vi "流程写入.vi"(10 "简易流程路径":path, 11 "添加的路径":path caption="测试流程路径") -> ()   [LabVIEW 2016, in "斯坦道总氮.lvlib"]
uses:
  <vilib>/Utility/miscctls.llb/LVPointTypeDef.ctl
panel:
  in  "选项卡控件":enum32{"测试流程", "简易流程"}(tab)
  in  "一键写入":bool
  in  "量程下拉列表":enum16{"低量程", "高量程"}(ring)
  in  "测量模式":T1(ring)
  in  "简易流程":u16(ring)
  in  "一键写入 2":bool=TRUE
  in  "关闭":bool
  out "字符串":string
  in  "写入":bool
  in  "参数下拉列表":u16(ring)
  # "请选择要写入的流程"
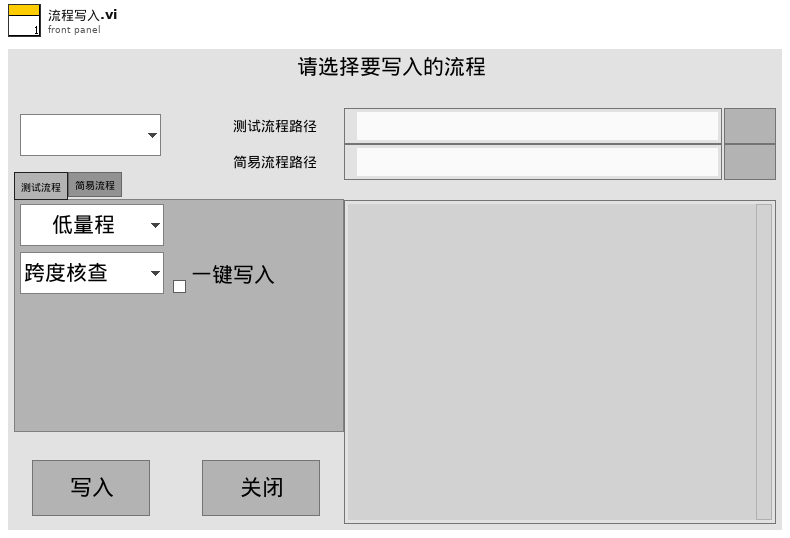
[diagram p1: front panel]
types:
  T1 = enum16{"跨度核查", "水样测量", "零点核查", "标样核查", "加标回收", "快捷测试", "空白校准", "标样校准"}
  T2 = typedef "LVPointTypeDef.ctl" = cluster{"Horizontal":i16, "Vertical":i16}
  T3 = typedef "LVStringsAndValuesArrayTypeDef_U16.ctl" = cluster{"String":string, "Value":u16}[]
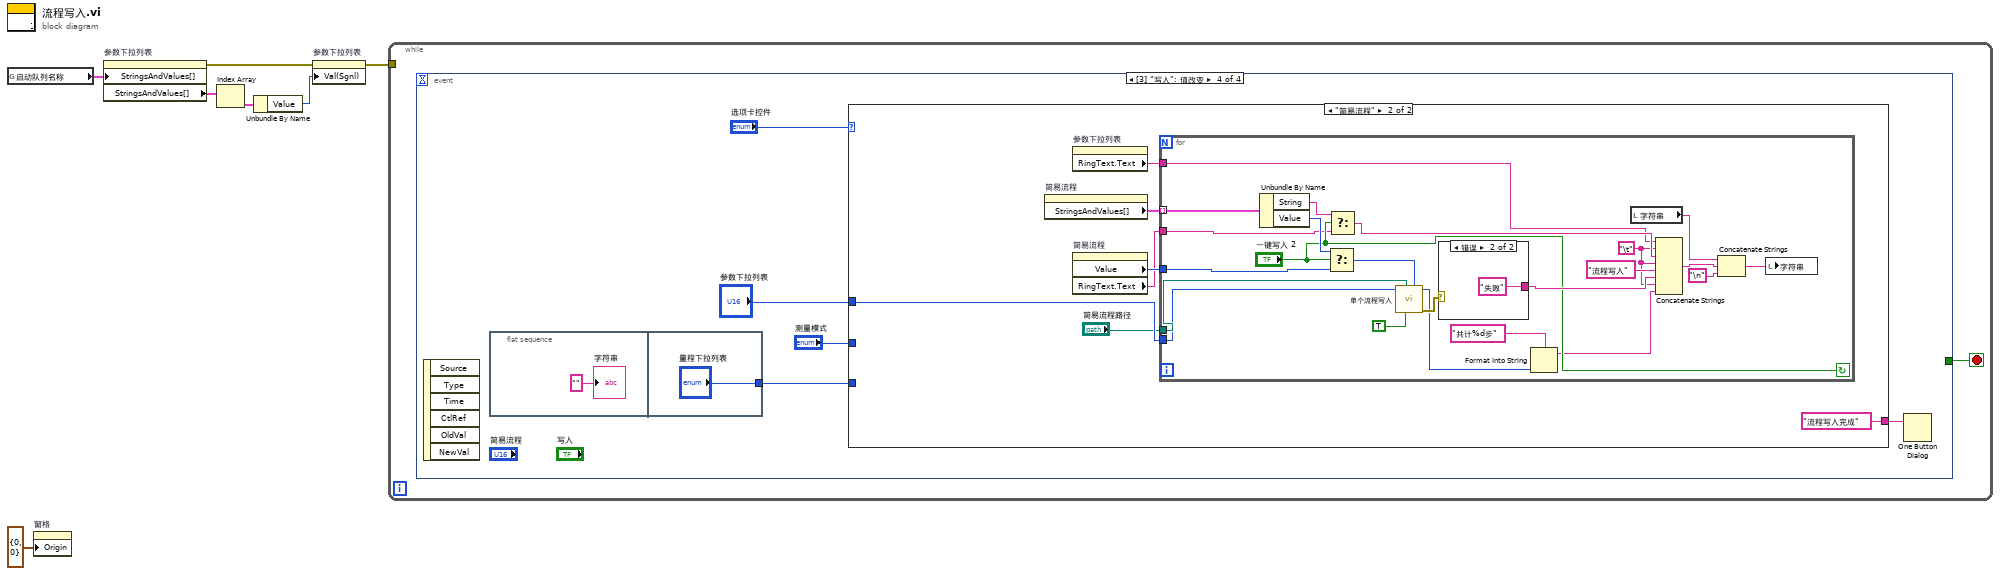
[diagram p0: block diagram]
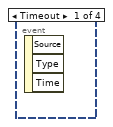
[diagram p2: hidden frame]
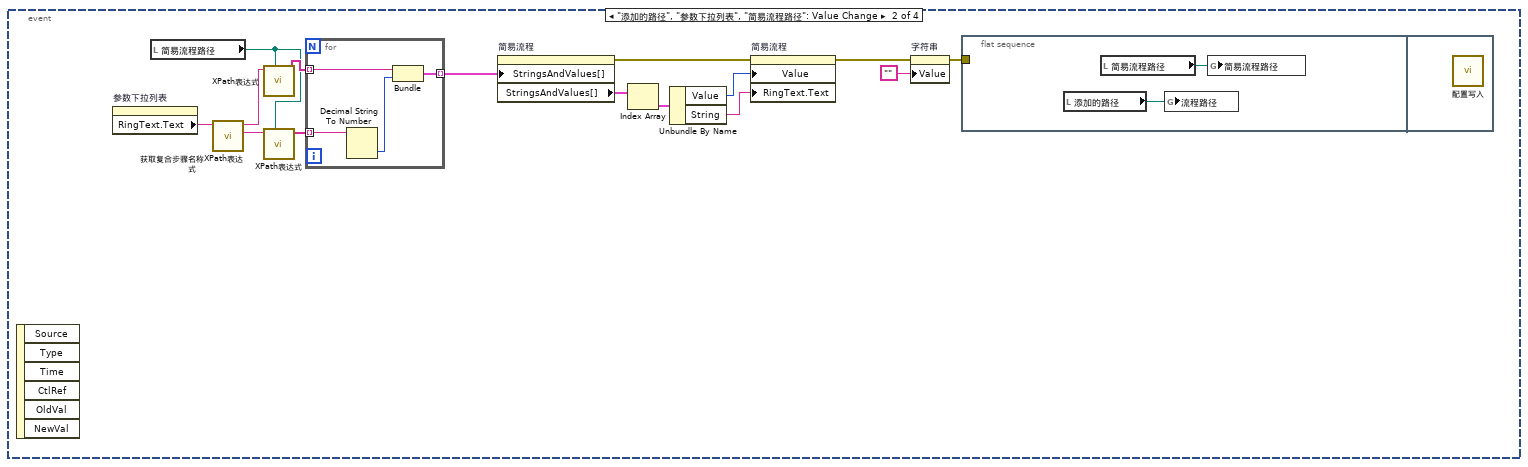
[diagram p3: hidden frame]
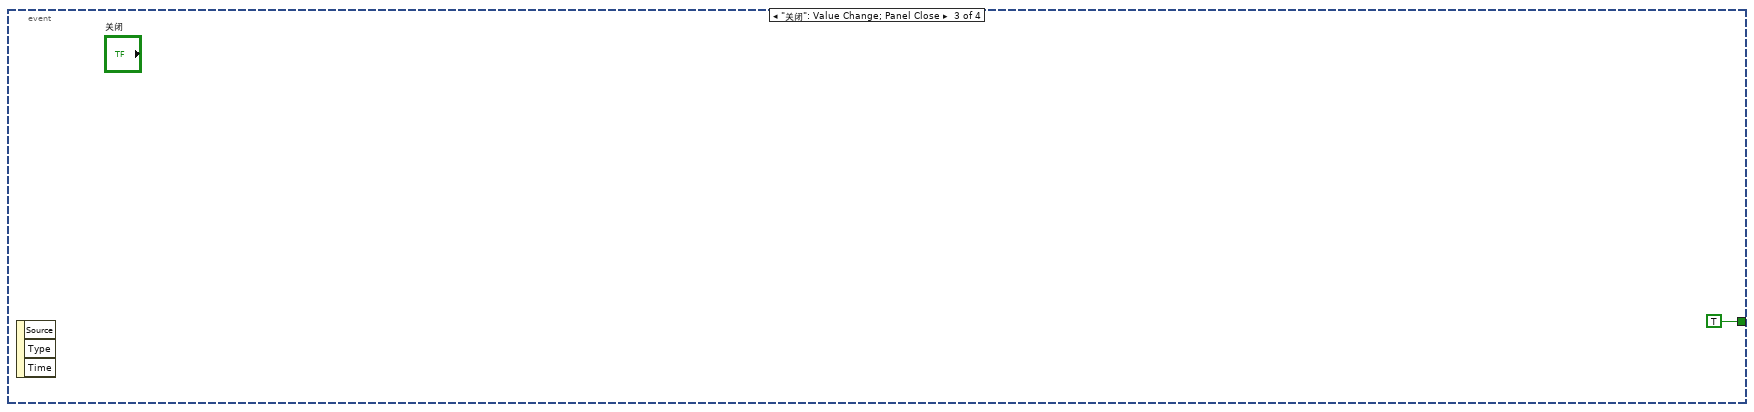
[diagram p4: hidden frame]
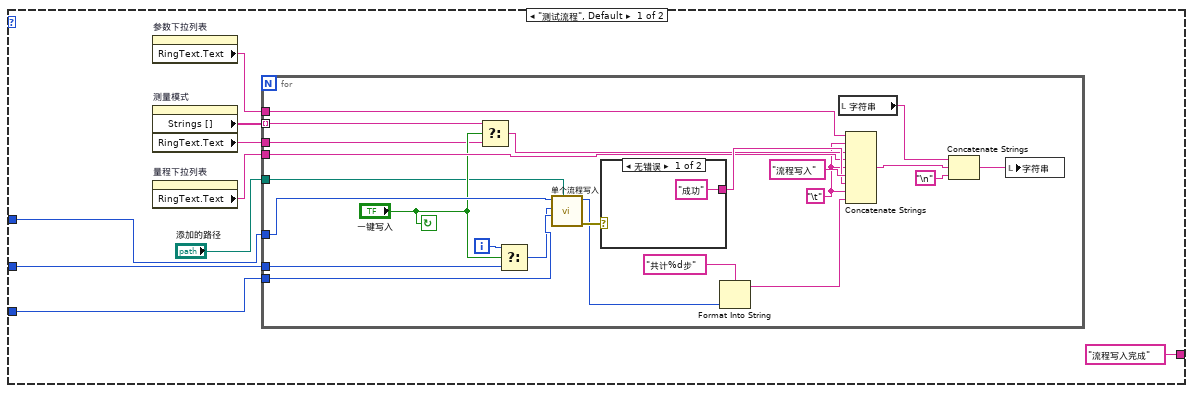
[diagram p5: hidden frame]
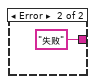
[diagram p6: hidden frame]
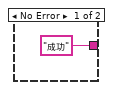
[diagram p7: hidden frame]
diagram:
  n1 = global read "总磷总氮断电保存全局变量.vi" "启动队列名称"() -> (w6:cluster{"String":string, "Value":u16}[])
  n2 = property on="窗格" class="Pane"("Origin"=T2 {"Horizontal"=0, "Vertical"=0} ("原点")) -> ()  [unwired: 2 in, 2 out]
  n3 = property on="参数下拉列表" class="Ring (严格)"("StringsAndValues[]"=w6) -> (error out=w5:errorcluster, "StringsAndValues[]"=w4:T3)  [unwired: 2 in, 1 out]
  n4 = Index Array(array=w4) -> (element=w3:cluster{"String":string, "Value":u16})  [unwired: 1 in]
  n5 = Unbundle By Name(w3) -> ("Value"=w2:u16)
  n6 = property on="参数下拉列表" class="Ring (严格)"(error in=w5, "Val(Sgnl)"=w2) -> (error out=w1:errorcluster)  [unwired: 1 in, 1 out]
  n7 = while {
    tunnel: w1 -> [_]
    stop <- w8 stop-if-true
    n8 = event shown="[3] \"写入\": 值改变" {
      selector: _ -> [_ _ _ _]
      dyn-events: _ -> [_ _ _ _]
      timeout: _ -> [_ _ _ _]
      tunnel: [_ _ TRUE _] -> w8
      event Timeout {
        n9 = event-data() -> ()  [unwired: 1 in, 3 out]
      }
      event "添加的路径", "参数下拉列表", "简易流程路径": Value Change {
        n10 = event-data() -> ()  [unwired: 1 in, 6 out]
        n11 = property on="参数下拉列表" class="Ring (严格)"() -> ("RingText.Text"=w22:string)  [unwired: 2 in, 2 out]
        n12 = local read "简易流程路径"() -> (w16:path)
        n13 = call "获取复合步骤名称XPath表达式.vi"("查询参数"=w22) -> ("FlowId"=w21:string, "name"=w23:string)  [unwired: 9 in]
        n14 = call "XPath表达式.vi"("添加的路径"=w16, "XPath expression"=w23) -> ("数组"=w20:string[])  [unwired: 9 in]
        n15 = call "XPath表达式.vi"("添加的路径"=w16, "XPath expression"=w21) -> ("数组"=w19:string[])  [unwired: 9 in]
        n16 = for {
          tunnel: w20 -> [w29] mode=indexing
          tunnel: w19 -> [w28] mode=indexing
          tunnel: [w26] -> w18 mode=indexing
          n17 = Decimal String To Number(string=w28) -> (number=w27:i32)  [unwired: 2 in, 1 out]
          n18 = Bundle("node text"=w29, w27) -> (w26:cluster{"node text":string, i32})  [unwired: 1 in]
        }
        n19 = property on="简易流程" class="Ring (严格)"("StringsAndValues[]"=w18) -> (error out=w15:errorcluster, "StringsAndValues[]"=w13:T3)  [unwired: 2 in, 1 out]
        n20 = Index Array(array=w13) -> (element=w12:cluster{"String":string, "Value":u16})  [unwired: 1 in]
        n21 = Unbundle By Name(w12) -> ("Value"=w11:u16, "String"=w9:string)
        n22 = property on="简易流程" class="Ring (严格)"(error in=w15, "Value"=w11, "RingText.Text"=w9) -> (error out=w14:errorcluster)  [unwired: 1 in, 1 out]
        n23 = property on="字符串" class="Str"(error in=w14, "Value"="") -> (error out=w10:errorcluster)  [unwired: 1 in, 1 out]
        n24 = flat-sequence {
          tunnel: w10 -> [_]
          frame #0 {
            n25 = local read "添加的路径"() -> (w24:path)
            n26 = local read "简易流程路径"() -> (w25:path)
            n27 = global write "总磷总氮断电保存全局变量.vi" "流程路径"(w24) -> ()
            n28 = global write "总磷总氮断电保存全局变量.vi" "简易流程路径"(w25) -> ()
          }
          frame #1 {
            n29 = call "配置写入.vi"() -> ()  [unwired: 11 in, 1 out]
          }
        }
      }
      event "关闭": Value Change; Panel Close {
        n30 = event-data() -> ()  [unwired: 1 in, 3 out]
      }
      event "写入": Value Change {
        n31 = event-data() -> ()  [unwired: 1 in, 6 out]
        n32 = flat-sequence {
          tunnel: ["量程下拉列表"] -> w34
          frame #0 {
            "字符串" <- ""
          }
          frame #1 {
          }
        }
        n33 = case shown="\"简易流程\"" "选项卡控件" {
          tunnel: "参数下拉列表" -> [w42 w76]
          tunnel: w34 -> [w43 _]
          tunnel: ["流程写入完成" ("消息") "流程写入完成" ("消息")] -> w32
          tunnel: "测量模式" -> [w40 _]
          frame "测试流程", Default {
            n34 = property on="参数下拉列表" class="Ring (严格)"() -> ("RingText.Text"=w37:string)  [unwired: 2 in, 2 out]
            n35 = property on="测量模式" class="Enum (严格)"() -> ("Strings []"=w41:string[], "RingText.Text"=w38:string)  [unwired: 2 in, 2 out]
            n36 = property on="量程下拉列表" class="Enum (严格)"() -> ("RingText.Text"=w39:string)  [unwired: 2 in, 2 out]
            n37 = for {
              tunnel: w43 -> [w60]
              tunnel: w42 -> [w58]
              tunnel: w41 -> [w53] mode=indexing
              tunnel: w40 -> [w57]
              tunnel: w39 -> [w55]
              tunnel: w38 -> [w52]
              tunnel: "添加的路径" -> [w50]
              tunnel: w37 -> [w49]
              i -> [w59]
              stop <- "一键写入" continue-if-true
              w45 = "\t"
              n38 = Select(t=w53, s="一键写入", f=w52) -> (s? t:f=w51:string)
              n39 = Select(t=w59, s="一键写入", f=w57) -> (s? t:f=w56:i32)
              n40 = call "单个流程写入.vi"("添加的路径"=w50, "量程"=w60, "测量模式"=w56, "测量参数"=w58) -> ("error out"=w67:errorcluster, "步数"=w48:i32)  [unwired: 6 in]
              n41 = case shown="无错误" w67 {
                tunnel: ["成功" "失败"] -> w64
                frame No Error {
                }
                frame Error {
                }
              }
              n42 = Format Into String(format string="共计%d步" ("格式字符串"), w48) -> (resulting string=w46:string)  [unwired: 2 in, 1 out]
              n43 = local read "字符串"() -> (w66:string)
              n44 = Concatenate Strings(w49, w45, w51, w55, w45, "流程写入", w64, w45, w46) -> (w63:string)
              n45 = Concatenate Strings(w66, w63, "\n") -> (w61:string)
              n46 = local write "字符串"(w61) -> ()
            }
          }
          frame "简易流程" {
            n47 = property on="简易流程" class="Ring (严格)"() -> ("StringsAndValues[]"=w75:T3)  [unwired: 2 in, 2 out]
            n48 = property on="参数下拉列表" class="Ring (严格)"() -> ("RingText.Text"=w70:string)  [unwired: 2 in, 2 out]
            n49 = property on="简易流程" class="Ring (严格)"() -> ("Value"=w73:u16, "RingText.Text"=w72:string)  [unwired: 2 in, 2 out]
            n50 = for {
              tunnel: w75 -> [w89] mode=indexing
              tunnel: "简易流程路径" -> [w92]
              tunnel: w76 -> [w91]
              tunnel: w73 -> [w86]
              tunnel: w72 -> [w83]
              tunnel: w70 -> [w77]
              stop <- "一键写入 2" continue-if-true
              w78 = "\t"
              n51 = Unbundle By Name(w89) -> ("String"=w84:string, "Value"=w88:u16)
              n52 = Select(t=w88, s="一键写入 2", f=w86) -> (s? t:f=w87:u16)
              n53 = Select(t=w84, s="一键写入 2", f=w83) -> (s? t:f=w82:string)
              n54 = call "单个流程写入.vi"("简易流程Id"=w87, "是否是简易流程"=TRUE, "添加的路径"=w92, "测量参数"=w91) -> ("error out"=w99:errorcluster, "步数"=w81:i32)  [unwired: 6 in]
              n55 = case shown="错误" w99 {
                tunnel: ["成功" "失败"] -> w96
                frame No Error {
                }
                frame Error {
                }
              }
              n56 = Format Into String(format string="共计%d步" ("格式字符串"), w81) -> (resulting string=w79:string)  [unwired: 2 in, 1 out]
              n57 = local read "字符串"() -> (w98:string)
              n58 = Concatenate Strings(w77, w78, w82, w78, "流程写入", w96, w78, w79) -> (w95:string)
              n59 = Concatenate Strings(w98, w95, "\n") -> (w93:string)
              n60 = local write "字符串"(w93) -> ()
            }
          }
        }
        n61 = One Button Dialog(message=w32) -> ()  [unwired: 1 in, 1 out]
      }
    }
  }
